vi "GetRebootLogFile.vi"(7 "LabVIEW Web Service Request":refnum<class "Web Request.lvclass">) -> ()   [LabVIEW 2017]
uses:
  <vilib>/wsapi/Web Request.lvclass
  <vilib>/addons/InsightCM/Utilities/GlobalConfiguration/GlobalConfiguration.lvlib
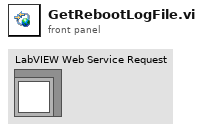
[diagram p1: front panel]
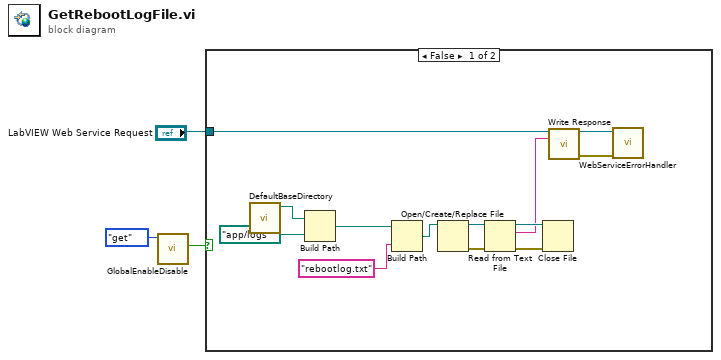
[diagram p0: block diagram]
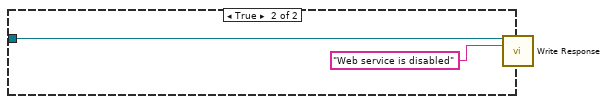
[diagram p2: hidden frame]
diagram:
  n1 = call "GlobalEnableDisable.vi"("action"=enum16{"init", "set", "get"}."get") -> ("DisableDeviceWebService"=w3:bool)  [unwired: 10 in]
  n2 = case shown="False" w3 {
    tunnel: "LabVIEW Web Service Request" -> [w12 w18]
    frame False {
      n3 = call <vilib>:"DefaultBaseDirectory.vi"() -> ("base directory"=w14:path)  [unwired: 11 in]
      n4 = Build Path(base path=w14, name or relative path=path "app/logs" ("base directory")) -> (appended path=w6:path)
      n5 = Build Path(base path=w6, name or relative path="rebootlog.txt") -> (appended path=w7:path)
      n6 = Open/Create/Replace File(file path (use dialog)=w7) -> (refnum out=w11:refnum<file>, error out=w9:errorcluster)  [unwired: 5 in, 1 out]
      n7 = Read from Text File(file (use dialog)=w11, error in=w9) -> (refnum out=w10:refnum<file>, text=w4:string, error out=w8:errorcluster)  [unwired: 2 in, 1 out]
      n8 = Close File(refnum=w10, error in=w8) -> ()  [unwired: 2 out]
      n9 = call <vilib>:"Write Response.vi"("LabVIEW Web Service Request"=w12, "response string"=w4) -> ("LabVIEW Web Service Request out"=w16:refnum<class "Web Request.lvclass">, "error out"=w15:errorcluster)  [unwired: 12 in]
      n10 = call "WebServiceErrorHandler.vi"("LabVIEW Web Service Request"=w16, "error in (no error)"=w15) -> ()  [unwired: 12 in, 2 out]
    }
    frame True {
      n11 = call <vilib>:"Write Response.vi"("LabVIEW Web Service Request"=w18, "response string"="Web service is disabled") -> ()  [unwired: 12 in, 2 out]
    }
  }
